vi "FRA example-AndreTec-2.vi"() -> ()   [LabVIEW 2014]
doc: "André Romero - 2016\nandretec@ifsc.usp.br\nIFSC - USP"
uses:
  <vilib>/Analysis/Matrix/Datatypes/RealMatrix.ctl
  C:/UserLabs/Andre/Nova-Autolab/Labview/Autolab SDK 1.11/EcoChemie.Autolab.Sdk.dll
  EcoChemie.Autolab.Sdk.dll
  <vilib>/Instr/_visa.llb/VISA Configure Serial Port (Instr).vi
  Global 1.vi
  <vilib>/Utility/file.llb/Write To Spreadsheet File (DBL).vi
  <vilib>/Analysis/Matrix/NI_Matrix.lvlib
panel:
  out "IsMeasuring":bool
  in  "Hardware Setup File":path
  in  "Embedded Exe File":path
  out "Graph Z2":cluster{"Y":dbl[], "-Z''":dbl[]}(graph)
  out "Graph Z":cluster{"Y":dbl[], "Z'":dbl[]}(graph)
  out "Bode phase":cluster{dbl[], dbl[]}(graph)
  out "Bode Z":cluster{dbl[], dbl[]}(graph)
  out "Magnitude Z":dbl[](array[numeric])
  out "Frequency 2":dbl[](array[numeric])
  out "Phase":dbl[](array[numeric])
  out "Frequency":dbl[](array[numeric])
  in  "Warning":string="Wait !!!! Instrument is initializing ...."
  in  "Start Measurement":bool
  out "Sensor":i32=1
  out "error out":errorcluster
  out "VISA resource name out":refnum<visa-resource-name>="ASRL3::INSTR"
  in  "N. Sensors":i32=3 min=1 max=8
  out "Points":i32=478
  in  "Abort":bool
  out "Measurement active":bool
  out "Blacklisted Commands detected":bool
  in  "Load Procedure (.nox)":path=path "C:/Users/user/Documents/My Procedures 1.11/Procedures/FRA lorenzo.nox"
  out "Autolab Connected":bool=TRUE
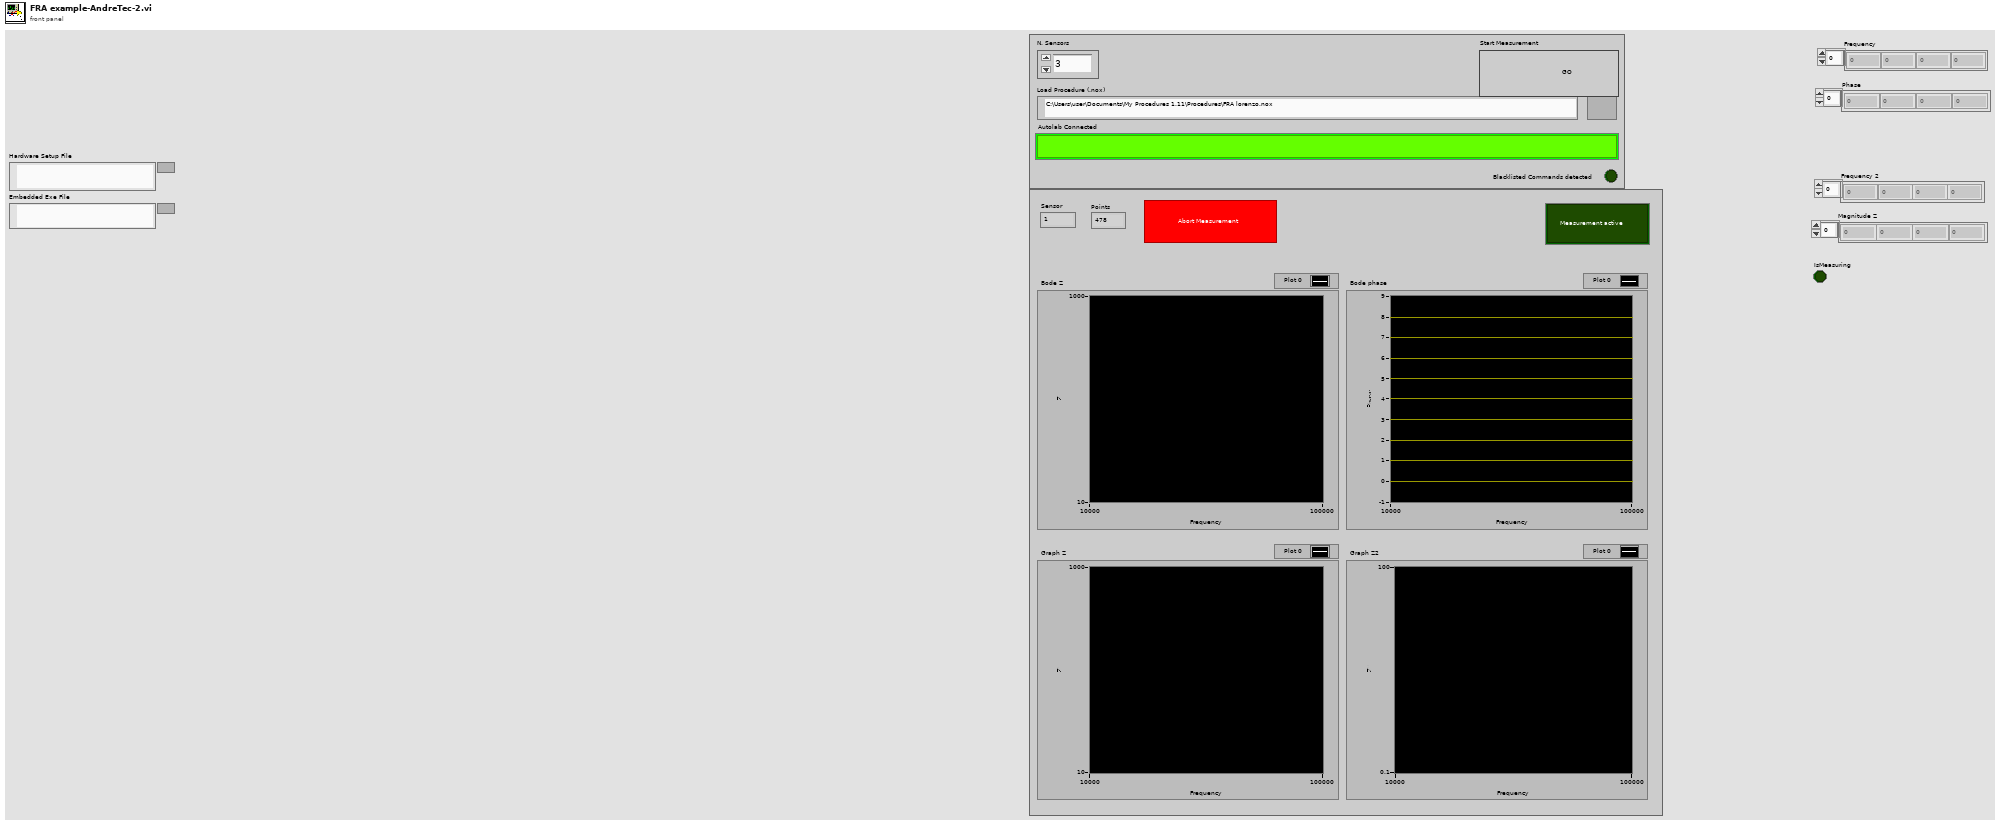
[diagram p1: front panel]
types:
  T1 = typedef "NI_Matrix.lvlib/RealMatrix.ctl" = dbl[][]
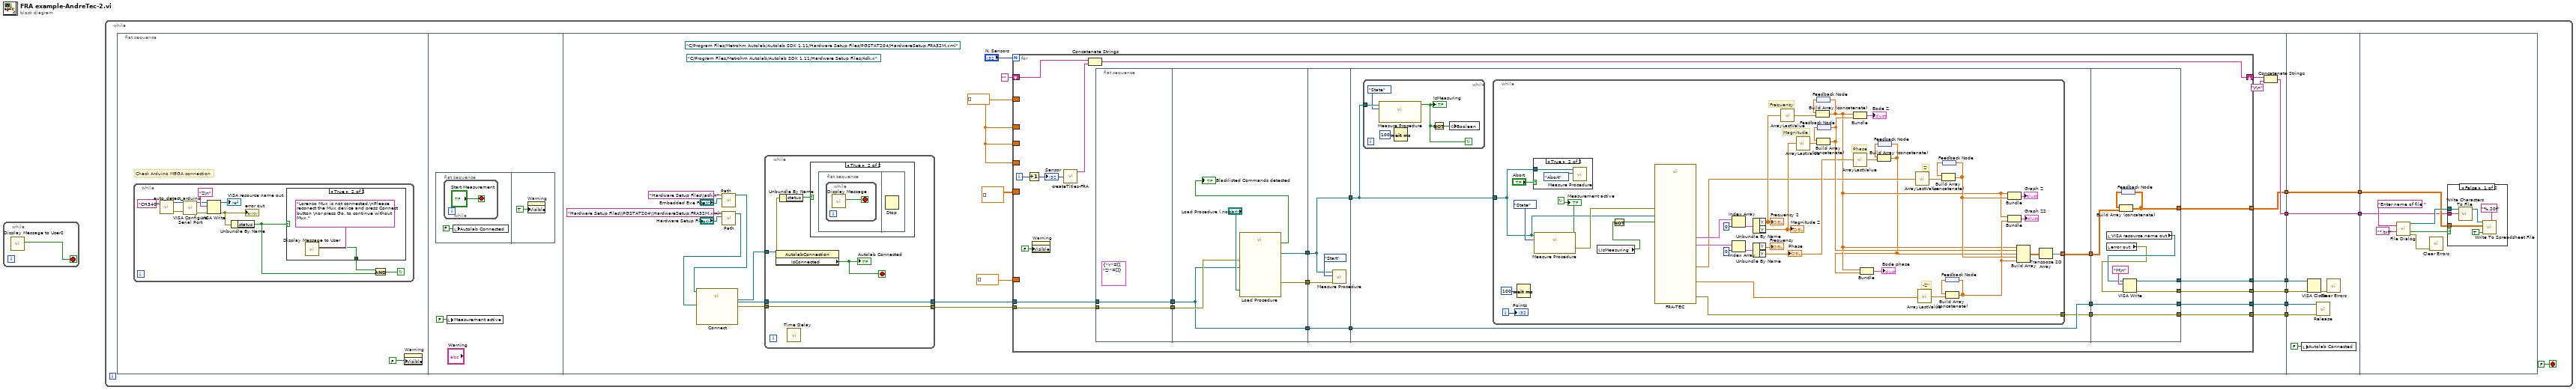
[diagram p0: block diagram]
diagram:
  n1 = while {
    stop <- w1 stop-if-true
    n2 = call "Display Message to User2"() -> ("OK"=w1:bool)  [unwired: 10 in, 1 out]
  }
  n3 = while {
    stop <- FALSE stop-if-true
    n4 = flat-sequence {
      tunnel: [w37] -> w9
      tunnel: [w43] -> w7
      tunnel: [w41] -> w5
      tunnel: [w40] -> w4
      tunnel: [w39] -> w3
      tunnel: [w38] -> w2
      tunnel: w9 -> [w166]
      tunnel: [w166] -> w8
      tunnel: w7 -> [w165]
      tunnel: [w165] -> w6
      tunnel: w5 -> [w162]
      tunnel: w4 -> [w161]
      tunnel: w3 -> [w160]
      tunnel: w2 -> [w159]
      tunnel: w8 -> [w170]
      tunnel: w6 -> [w169]
      frame #0 {
        # "Check Arduino MEGA connection"
        n5 = while {
          stop <- w14 continue-if-true
          n6 = call "auto_detect_arduino.vi"("instr name"="CH340") -> ("VISA resource name"=w22:refnum<visa-resource-name>, "error out"=w15:errorcluster)  [unwired: 1 in, 1 out]
          n7 = call-poly "VISA Configure Serial Port"("VISA resource name"=w22, "error in (no error)"=w15) -> ("VISA resource name out"=w19:refnum<visa-resource-name>, "error out"=w18:errorcluster)  [unwired: 7 in, 5 out]
          n8 = VISA Write(VISA resource name=w19, write buffer="Z\n" ("Command"), error in (no error)=w18) -> (VISA resource name out=→"VISA resource name out":refnum<visa-resource-name>, error out=w16:errorcluster)  [unwired: 1 out]
          "error out" <- w16
          n9 = Unbundle By Name(w16) -> ("status"=w13:bool)
          n10 = case shown="True" w13 {
            tunnel: [_ w23] -> w12
            frame False {
            }
            frame True {
              n11 = call "Display Message to User"("Message"="Lorenzo Mux is not connected.\nPlease reconect the Mux device and press Connect button \nor press Go, to continue without Mux.") -> ("Connect"=w23:bool)  [unwired: 9 in, 1 out]
            }
          }
          n12 = And(x=w12, y=w13) -> (x .and. y?=w14:bool)
        }
        n13 = property on="Warning" class="Str"("Visible"=FALSE) -> ()  [unwired: 2 in, 2 out]
      }
      frame #1 {
        n14 = flat-sequence {
          frame #0 {
            n15 = while {
              stop <- "Start Measurement" stop-if-true
            }
            n16 = local write "Autolab Connected"(FALSE ("Autolab Connected")) -> ()
          }
          frame #1 {
            n17 = property on="Warning" class="Str"("Visible"=TRUE) -> ()  [unwired: 2 in, 2 out]
          }
        }
        n18 = local write "Measurement active"(FALSE ("Measurement active")) -> ()
      }
      frame #2 {
        w30 = dbl[] []
        (unwired) path "C:/Program Files/Metrohm Autolab/Autolab SDK 1.11/Hardware Setup Files/Adk.x" ("Embedded Exe File")
        (unwired) path "C:/Program Files/Metrohm Autolab/Autolab SDK 1.11/Hardware Setup Files/PGSTAT204/HardwareSetup.FRA32M.xml" ("Hardware Setup File")
        n19 = call "Path.vi"("File"="Embedded Exe File", "name or relative path"="Hardware Setup Files\\adk.x") -> ("appended path"=w32:path)  [unwired: 9 in]
        n20 = call "Path.vi"("File"="Hardware Setup File", "name or relative path"="Hardware Setup Files\\PGSTAT204\\HardwareSetup.FRA32M.xml") -> ("appended path"=w31:path)  [unwired: 9 in]
        n21 = call "Connect.vi"("Embedded Exe File"=w32, "Hardware Setup File"=w31) -> ("AutolabConnection"=w52:refnum<k24>, "instrument"=w51:refnum<k24>, "error out"=w49:errorcluster)  [unwired: 1 in, 10 out]
        n22 = while {
          tunnel: w52 -> [w156]
          tunnel: w51 -> [w153]
          tunnel: [w153] -> w50
          tunnel: w49 -> [w152]
          tunnel: [w152] -> w48
          stop <- w157 stop-if-true
          n23 = property class="AutolabConnection"(reference=w156) -> (error out=w154:errorcluster, "IsConnected"=w157:bool)  [unwired: 1 in, 1 out]
          "Autolab Connected" <- w157
          n24 = Unbundle By Name(w154) -> ("status"=w155:bool)
          n25 = call "Time Delay"() -> ()  [unwired: 2 in, 10 out]
          n26 = case shown="True" w155 {
            frame False {
            }
            frame True {
              n27 = flat-sequence {
                frame #0 {
                  n28 = while {
                    stop <- w158 stop-if-true
                    n29 = call "Display Message"() -> ("OK"=w158:bool)  [unwired: 10 in, 1 out]
                  }
                }
                frame #1 {
                  n30 = Stop() -> ()  [unwired: 1 in]
                }
              }
            }
          }
        }
        n31 = for {
          N: "N. Sensors" -> [_]
          tunnel: [w70] -> w41
          tunnel: [w69] -> w40
          tunnel: [w68] -> w39
          tunnel: [w67] -> w38
          tunnel: w48 -> [w66]
          tunnel: w50 -> [w65]
          border: T1 [] ("Real Matrix") -> [_]
          shift-right: [w59] -> w44
          shift-left: "" -> [w61]
          tunnel: [w57] -> w37
          border: w30 -> [_]
          border: w30 -> [_]
          border: w30 -> [_]
          border: w30 -> [_]
          border: dbl[] [] -> [_]
          i -> [w63]
          n32 = Increment(x=w63) -> (x+1=w58:i32)
          "Sensor" <- w58
          n33 = property on="Warning" class="Str"("Visible"=FALSE) -> ()  [unwired: 2 in, 2 out]
          n34 = call "createTitles-FRA.vi"("Sensor Number"=w58) -> ("String"=w60:string)  [unwired: 10 in]
          n35 = Concatenate Strings(w61, w60) -> (w59:string)
          n36 = flat-sequence {
            tunnel: w66 -> [w76]
            tunnel: w65 -> [w77]
            tunnel: [w77] -> w56
            tunnel: [w76] -> w55
            tunnel: [w81] -> w75
            tunnel: [w80] -> w74
            tunnel: [w78] -> w73
            tunnel: w56 -> [w78]
            tunnel: w55 -> [w79]
            tunnel: w75 -> [w85]
            tunnel: w74 -> [w86]
            tunnel: [w85] -> w54
            tunnel: [w84] -> w53
            tunnel: w73 -> [w84]
            tunnel: w54 -> [w88]
            tunnel: w53 -> [w91]
            tunnel: [w91] -> w72
            tunnel: [w89] -> w71
            tunnel: [w90] -> w64
            tunnel: w72 -> [w151]
            tunnel: w71 -> [w150]
            tunnel: [w151] -> w70
            tunnel: [w150] -> w69
            tunnel: [w146] -> w68
            tunnel: [w145] -> w67
            tunnel: w64 -> [w143]
            tunnel: [w142] -> w57
            frame #0 {
              (unwired) cluster{"Y":dbl[], "Z'":dbl[]} {"Y"=[], "Z'"=[]} ("Graph Z")
            }
            frame #1 {
              n37 = call "Load Procedure.vi"("error in (no error)"=w79, "Procedure"="Load Procedure (.nox)", "Instrument"=w78) -> ("error out"=w80:errorcluster, "Contains"=→"Blacklisted Commands detected":bool, "LoadProcedure"=w81:refnum<k24>)  [unwired: 6 out]
            }
            frame #2 {
              n38 = call "Measure Procedure.vi"("error in"=w86, "Request for procedure"=enum16{"State", "Save", "Abort", "Start"}."Start", "LoadProcedure"=w85) -> ()  [unwired: 1 in, 8 out]
            }
            frame #3 {
              n39 = while {
                tunnel: w88 -> [w96]
                stop <- w93 continue-if-true
                n40 = call "Measure Procedure.vi"("Request for procedure"=enum16{"State", "Save", "Abort", "Start"}."State", "LoadProcedure"=w96) -> ("IsMeasuring"=w93:bool)  [unwired: 2 in, 7 out]
                "IsMeasuring" <- w93
                n41 = Wait (ms)(milliseconds to wait=u32 100) -> ()  [unwired: 1 out]
                n42 = Not(x=w93) -> (.not. x?=w92:bool)
                n43 = global write "Global 1.vi" "Boolean"(w92) -> ()
              }
              n44 = while {
                tunnel: w88 -> [w133]
                tunnel: [w136] -> w90
                tunnel: [w134] -> w89
                i -> [w137]
                stop <- w131 continue-if-true
                # "-Z''"
                # "Z'"
                # "Phase"
                # "Magnitude"
                # "Frequency"
                n45 = Wait (ms)(milliseconds to wait=u32 100) -> ()  [unwired: 1 out]
                n46 = case shown="True" "Abort" {
                  tunnel: w133 -> [_ w140]
                  frame False {
                  }
                  frame True {
                    n47 = call "Measure Procedure.vi"("Request for procedure"=enum16{"State", "Save", "Abort", "Start"}."Abort", "LoadProcedure"=w140) -> ()  [unwired: 2 in, 8 out]
                  }
                }
                n48 = call "Measure Procedure.vi"("Request for procedure"=enum16{"State", "Save", "Abort", "Start"}."State", "LoadProcedure"=w133) -> ("error out"=w135:errorcluster, "IsMeasuring"=w131:bool)  [unwired: 2 in, 6 out]
                "Measurement active" <- w131
                n49 = local read "IsMeasuring"() -> (w129:bool)
                n50 = Not(x=w129) -> (.not. x?=w130:bool)
                n51 = call "FRA-TEC.vi"("LoadProcedure"=w133, "stop"=w130, "error in"=w135) -> ("Bode phase"=w123:cluster{"Y":dbl[], "Y":dbl[]}[], "Bode Z"=w122:cluster{"Y":dbl[], "Y":dbl[]}[], "-Z''"=w103:dbl[], "Z'"=w105:dbl[], "error out"=w134:errorcluster)  [unwired: 15 in, 5 out]
                n52 = Index Array(array=w122, index=0) -> (element=w124:cluster{"Y":dbl[], "Y":dbl[]})
                n53 = Index Array(array=w123, index=0) -> (element=w126:cluster{"Y":dbl[], "Y":dbl[]})
                n54 = Unbundle By Name(w124) -> ("Y"=w119:dbl[], "Y"=w118:dbl[])
                "Frequency 2" <- w119
                "Magnitude Z" <- w118
                n55 = Unbundle By Name(w126) -> ("Y"=→"Frequency":dbl[], "Y"=w110:dbl[])
                "Phase" <- w110
                n56 = call "ArrayLastValue.vi"("Array In"=w119) -> ("Last value"=w116:dbl)
                n57 = call "ArrayLastValue.vi"("Array In"=w118) -> ("Last value"=w114:dbl)
                n58 = feedback #1() -> (w117:dbl[])
                n59 = Build Array (concatenate)(w117, w116) -> (w99:dbl[])
                n60 = feedback-in #1(w99) -> ()
                n61 = feedback #2() -> (w115:dbl[])
                n62 = Build Array (concatenate)(w115, w114) -> (w112:dbl[])
                n63 = feedback-in #2(w112) -> ()
                n64 = Bundle(w99, w112) -> (→"Bode Z":cluster{dbl[], dbl[]})  [unwired: 1 in]
                n65 = call "ArrayLastValue.vi"("Array In"=w110) -> ("Last value"=w108:dbl)
                n66 = feedback #3() -> (w109:dbl[])
                n67 = Build Array (concatenate)(w109, w108) -> (w98:dbl[])
                n68 = Bundle(w99, w98) -> (→"Bode phase":cluster{dbl[], dbl[]})  [unwired: 1 in]
                n69 = feedback-in #3(w98) -> ()
                n70 = call "ArrayLastValue.vi"("Array In"=w105) -> ("Last value"=w107:dbl)
                n71 = call "ArrayLastValue.vi"("Array In"=w103) -> ("Last value"=w102:dbl)
                n72 = feedback #4() -> (w106:dbl[])
                n73 = Build Array (concatenate)(w106, w107) -> (w104:dbl[])
                n74 = feedback-in #4(w104) -> ()
                n75 = feedback #5() -> (w101:dbl[])
                n76 = Build Array (concatenate)(w101, w102) -> (w100:dbl[])
                n77 = feedback-in #5(w100) -> ()
                n78 = Bundle(w99, w104) -> (→"Graph Z":cluster{dbl[], dbl[]})  [unwired: 1 in]
                n79 = Bundle(w99, w100) -> (→"Graph Z2":cluster{dbl[], dbl[]})  [unwired: 1 in]
                n80 = Build Array(w99, w112, w98, w104, w100) -> (w128:dbl[][])
                n81 = Transpose 2D Array(2D array=w128) -> (transposed array=w136:dbl[][])
                "Points" <- w137
              }
            }
            frame #4 {
              n82 = local read "error out"() -> (w147:errorcluster)
              n83 = local read "VISA resource name out"() -> (w148:refnum<visa-resource-name>)
              n84 = feedback #6() -> (w144:T1)
              n85 = Build Array (concatenate)(w144, w143) -> (w142:T1)
              n86 = feedback-in #6(w142) -> ()
              n87 = VISA Write(VISA resource name=w148, write buffer="M\n" ("Command"), error in (no error)=w147) -> (VISA resource name out=w146:refnum<visa-resource-name>, error out=w145:errorcluster)  [unwired: 1 out]
            }
          }
        }
        n88 = Concatenate Strings(w44, "\r\n") -> (w43:string)
      }
      frame #3 {
        n89 = local write "Autolab Connected"(FALSE ("Autolab Connected")) -> ()
        n90 = VISA Close(VISA resource name=w160, error in (no error)=w159) -> (error out=w163:errorcluster)
        n91 = call "Release.vi"("error in (no error)"=w161, "Instrument"=w162) -> ()  [unwired: 1 in, 9 out]
        n92 = call <vilib>:"Clear Errors.vi"("error in (no error)"=w163) -> ()  [unwired: 5 in, 2 out]
      }
      frame #4 {
        n93 = call "File Dialog"("prompt"="Enter name of file ", "pattern (all files)"="*.txt") -> ("selected path"=w171:path, "cancelled"=w167:bool, "error out"=w168:errorcluster)  [unwired: 10 in, 1 out]
        n94 = call <vilib>:"Clear Errors.vi"("error in (no error)"=w168) -> ()  [unwired: 5 in, 2 out]
        n95 = case shown="False" w167 {
          tunnel: w171 -> [w179 _]
          tunnel: w170 -> [w176 _]
          tunnel: w169 -> [w175 _]
          frame False {
            n96 = call <vilib>:"Write Characters To File.vi"("character string"=w175, "file path (dialog if empty)"=w179) -> ("new file path (Not A Path if cancelled)"=w178:path)  [unwired: 3 in]
            n97 = call-poly <vilib>:"Write To Spreadsheet File.vi"("format (%.3f)"="%.20f", "append to file? (new file:F)"=TRUE, "2D data"=w176, "file path (dialog if empty)"=w178) -> ()  [unwired: 4 in, 1 out]
          }
          frame True {
          }
        }
      }
    }
  }
